vi "pl1000GetUnitInfo.vi"(8 "error in (no error)":errorcluster, 10 "Info":T1(ring), 11 "pl1000 handle":i16) -> (0 "error out":errorcluster, 2 "String":string, 3 "pl1000 handle out":i16)   [LabVIEW 2016, in "pl1000.lvlib"]
uses:
  pl1000.lvlib
  pl1000.dll
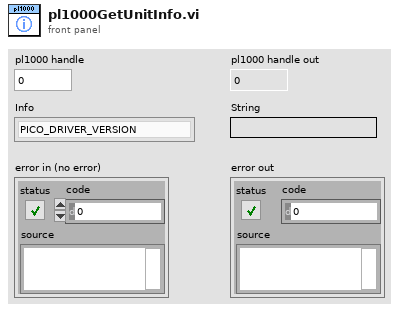
[diagram p1: front panel]
types:
  T1 = enum32{"PICO_DRIVER_VERSION ", "PICO_USB_VERSION", "PICO_HARDWARE_VERSION", "PICO_VARIANT_INFO", "PICO_BATCH_AND_SERIAL ", "PICO_CAL_DATE", "PICO_KERNEL_VERSION"}
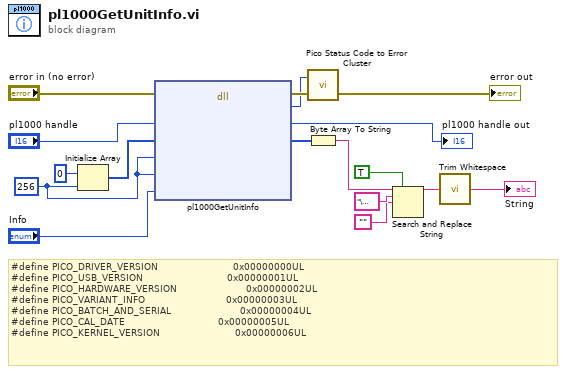
[diagram p0: block diagram]
diagram:
  w6 = 256 ("dimension size")
  # "#define\tPICO_DRIVER_VERSION                         0x00000000UL\n#define\tPICO_USB_VERSION                            0x00000001UL\n#define\tPICO_HARDWARE_VERSION                       0x00000002UL\n#define\tPICO_VARIANT_INFO                           0x00000003UL\n#define\tPICO_BATCH_AND_SERIAL                       0x00000004UL\n#define\tPICO_CAL_DATE                               0x00000005UL\n#define\tPICO_KERNEL_VERSION                         0x00000006UL"
  n1 = Initialize Array(u8 0 ("U8"), w6) -> (w7:u8[])
  n2 = dll-call lib="pl1000.dll" fn="pl1000GetUnitInfo"(error in="error in (no error)", "Handle"="pl1000 handle", "String"=w7, "StringLength"=w6, "RequiredSize"=w6, "PICO_INFO"="Info") -> (error out=w4:errorcluster, "status"=w3:u32, "Handle"=→"pl1000 handle out":i16, "String"=w11:u8[])  [unwired: 5 in, 1 out]
  n3 = call "Pico Status Code to Error Cluster.vi"("error in"=w4, "PICO_STATUS"=w3) -> ("error out"=→"error out":errorcluster)  [unwired: 1 in]
  n4 = Byte Array To String(unsigned byte array=w11) -> (string=w15:string)
  n5 = Search and Replace String(replace all?=TRUE ("replace all? (F)"), input string=w15, search string="\u0000", replace string="") -> (result string=w14:string)  [unwired: 4 in, 3 out]
  n6 = call <vilib>:"Trim Whitespace.vi"("string"=w14) -> ("trimmed string"=→"String":string)  [unwired: 1 in]
